vi "Make Suite from Test Case Path.vi"(8 "error in (no error)":errorcluster, 10 "Test Case":path) -> (0 "error out":errorcluster, 3 "LUnit Test Suite Out":refnum<class "LUnit Test Suite.lvclass">)   [LabVIEW 2020, in "Test Finder.lvclass"]
doc: "Produce a test suite including all test methods in a single test case class."
uses:
  LUnit Test Suite.lvclass
  LUnit Test Case.lvclass
  Test Finder.lvclass
  Test Finder.lvclass/Test Finder.ctl
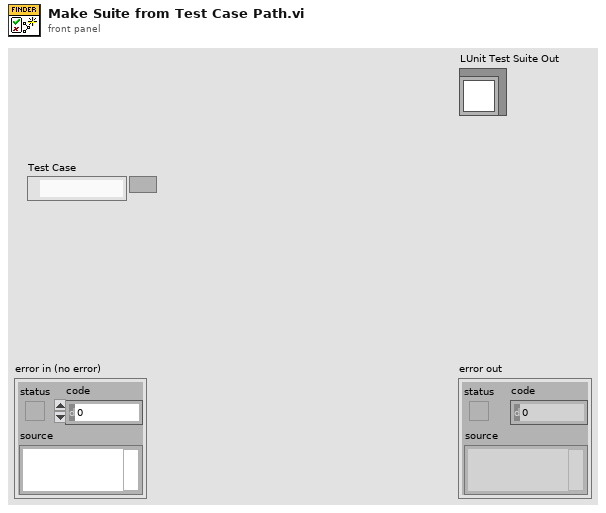
[diagram p1: front panel]
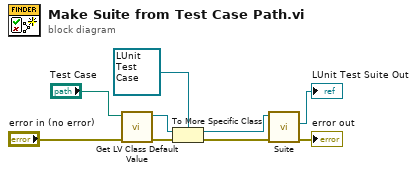
[diagram p0: block diagram]
diagram:
  n1 = call <vilib>:"Get LV Class Default Value.vi"("error in (no error)"="error in (no error)", "class path"="Test Case") -> ("error out"=w6:errorcluster, "object"=w7:refnum<class>)  [unwired: 8 in]
  n2 = To More Specific Class(target class=refnum<class "LUnit Test Case.lvclass"> refnum ("LUnit Test Case.lvclass"), reference=w7, error in=w6) -> (specific class reference=w4:refnum<class "LUnit Test Case.lvclass">, error out=w5:errorcluster)
  n3 = call-dynamic "Suite.vi"("error in (no error)"=w5, "LUnit Test Case In"=w4) -> ("error out"=→"error out":errorcluster, "LUnit Test Suite Out"=→"LUnit Test Suite Out":refnum<class "LUnit Test Suite.lvclass">)  [unwired: 7 in, 1 out]
